vi "main--example pop-up gif.vi"() -> ()   [LabVIEW 2021]
doc: "This VI will show a couple examples of loading images in as custom GIFs."
uses:
  <vilib>/addons/_TSC/TSC Pop-Up/Popup/message info--typedef.ctl
  Custom/GIF - One Button/GIF - One Button.lvclass
  <vilib>/addons/_TSC/TSC Pop-Up/Popup/Popup.lvclass
  user32.dll
panel:
  in  "Close":bool
  out "header":bool
  in  "danger":bool
  in  "happy-dance":bool
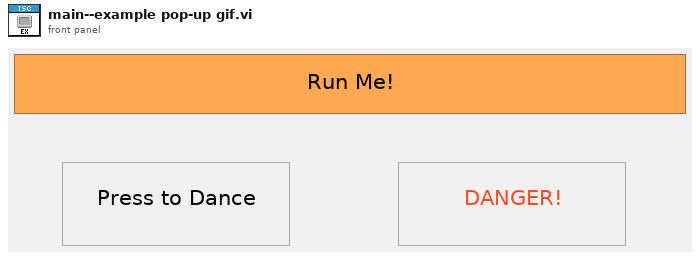
[diagram p1: front panel]
types:
  T1 = typedef "Pop-Up.lvlib/Popup.lvclass/message info--typedef.ctl" = cluster{"Message Height":i32, "Message Width":i32, "Message Location":enum16{"Top", "Bottom", "Right", "Left"}}
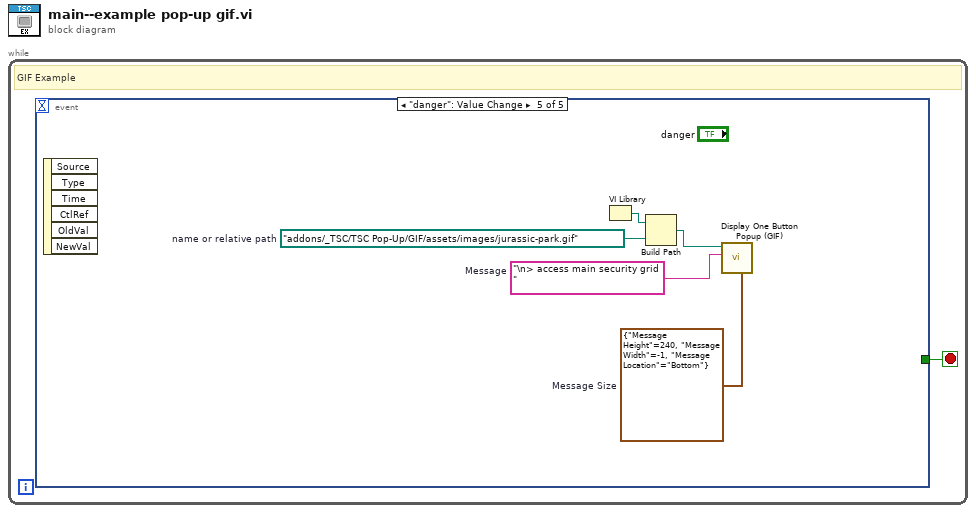
[diagram p0: block diagram]
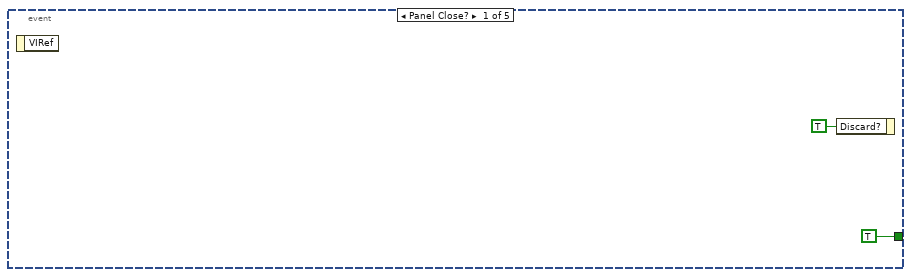
[diagram p2: hidden frame]
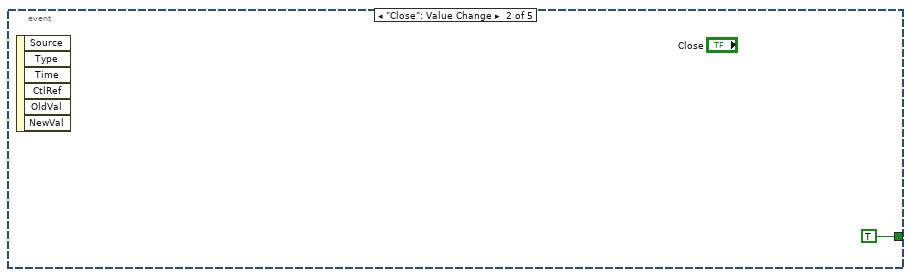
[diagram p3: hidden frame]
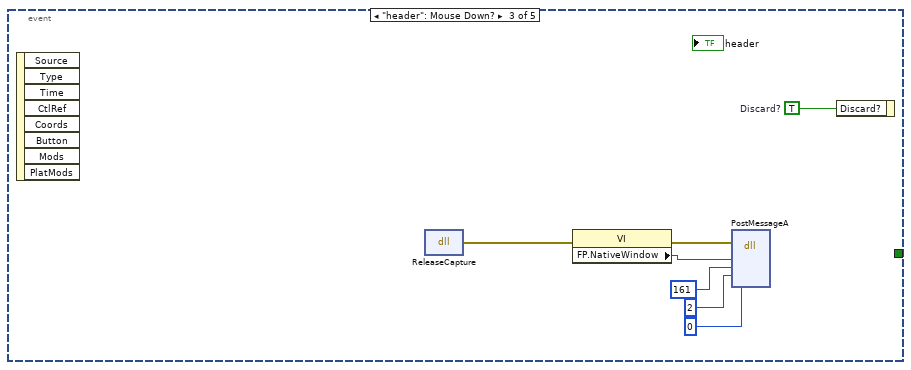
[diagram p4: hidden frame]
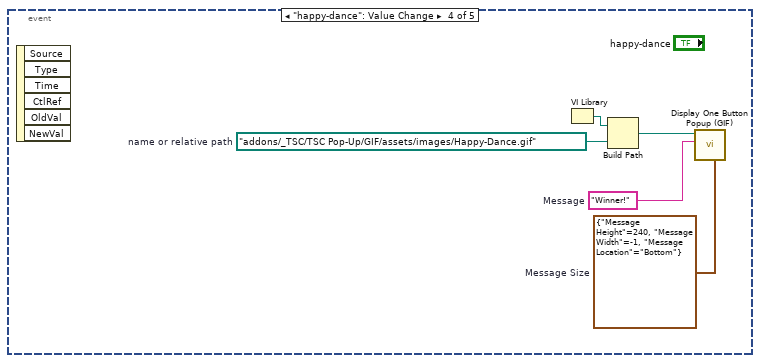
[diagram p5: hidden frame]
diagram:
  n1 = while {
    stop <- w1 stop-if-true
    # "GIF Example"
    n2 = event shown="[4] \"danger\": Value Change" {
      selector: _ -> [_ _ _ _ _]
      dyn-events: _ -> [_ _ _ _ _]
      timeout: _ -> [_ _ _ _ _]
      tunnel: [TRUE TRUE _ _ _] -> w1
      event Panel Close? {
        n3 = event-data() -> ()  [unwired: 1 in, 1 out]
        n4 = event-data("Discard?"=TRUE) -> ()  [unwired: 1 in, 1 out]
      }
      event "Close": Value Change {
        n5 = event-data() -> ()  [unwired: 1 in, 6 out]
      }
      event "header": Mouse Down? {
        w11 = TRUE  # Discard?
        n6 = event-data() -> ()  [unwired: 1 in, 8 out]
        n7 = dll-call lib="user32.dll" fn="ReleaseCapture"() -> (error out=w7:errorcluster)  [unwired: 4 in, 1 out]
        n8 = property class="VI"(error in=w7) -> (error out=w6:errorcluster, "FP.NativeWindow"=w5:u64)  [unwired: 1 in, 1 out]
        n9 = dll-call lib="user32.dll" fn="PostMessageA"(error in=w6, "hWnd"=w5, "Msg"=161, "wParam"=2, "lParam"=0) -> ()  [unwired: 7 in, 2 out]
        n10 = event-data("Discard?"=w11) -> ()  [unwired: 1 in, 1 out]
      }
      event "happy-dance": Value Change {
        w13 = path "addons/_TSC/TSC Pop-Up/GIF/assets/images/Happy-Dance.gif"  # name or relative path
        w15 = T1 {"Message Height"=240, "Message Width"=-1, "Message Location"=enum."Bottom"}  # Message Size
        w16 = "Winner!"  # Message
        n11 = event-data() -> ()  [unwired: 1 in, 6 out]
        n12 = VI Library() -> (path=w14:path)
        n13 = Build Path(base path=w14, name or relative path=w13) -> (appended path=w12:path)
        n14 = call "Display One Button Popup (GIF).vi"("Message Size"=w15, "Message"=w16, "Graphic"=w12) -> ()  [unwired: 8 in, 1 out]
      }
      event "danger": Value Change {
        w18 = path "addons/_TSC/TSC Pop-Up/GIF/assets/images/jurassic-park.gif"  # name or relative path
        w20 = T1 {"Message Height"=240, "Message Width"=-1, "Message Location"=enum."Bottom"}  # Message Size
        w21 = "\n> access main security grid "  # Message
        n15 = event-data() -> ()  [unwired: 1 in, 6 out]
        n16 = VI Library() -> (path=w19:path)
        n17 = Build Path(base path=w19, name or relative path=w18) -> (appended path=w17:path)
        n18 = call "Display One Button Popup (GIF).vi"("Message Size"=w20, "Message"=w21, "Graphic"=w17) -> ()  [unwired: 8 in, 1 out]
      }
    }
  }
